vi "ApplyIVIConfigurationStore.vi"(8 "error in (no error)":errorcluster, 11 "Path":path) -> (0 "error out":errorcluster)   [LabVIEW 2009]
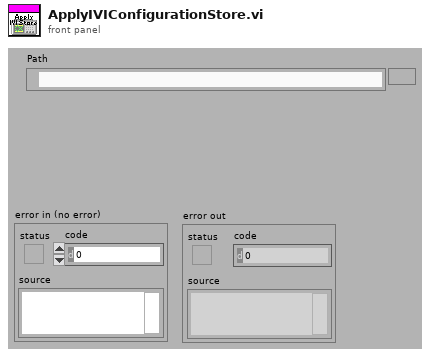
[diagram p1: front panel]
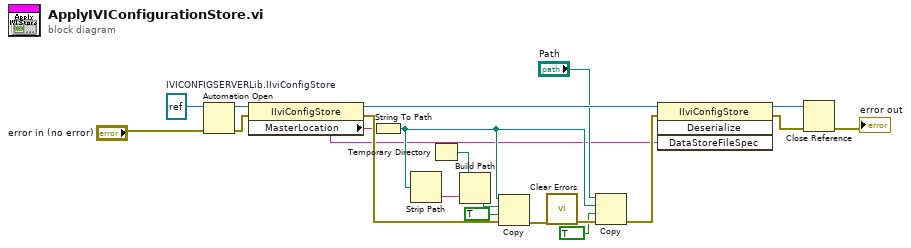
[diagram p0: block diagram]
diagram:
  w20 = refnum<k7> refnum  # IVICONFIGSERVERLib.IIviConfigStore
  n1 = Automation Open(error in (no error)="error in (no error)", Automation Refnum=w20) -> (Automation Refnum=w18:refnum<k7>, error out=w19:errorcluster)  [unwired: 2 out]
  n2 = property class="IIviConfigStore"(reference=w18, error in=w19) -> (reference out=w17:refnum<k7>, error out=w13:errorcluster, "MasterLocation"=w3:string)
  n3 = String To Path(string=w3) -> (path=w5:path)
  n4 = Strip Path(path=w5) -> (name=w15:string)  [unwired: 1 out]
  n5 = Temporary Directory() -> (w14:path)
  n6 = Build Path(base path=w14, name or relative path=w15) -> (appended path=w8:path)
  n7 = Copy(8:w13, 9:TRUE ("overwrite (F)"), 10:w8, 11:w5) -> (0:w16:errorcluster)  [unwired: 1 in, 2 out]
  n8 = call <vilib>:"Clear Errors.vi"("error in (no error)"=w16) -> ("error out"=w7:errorcluster)  [unwired: 6 in]
  n9 = Copy(8:w7, 9:TRUE ("overwrite (F)"), 10:w5, 11:"Path") -> (0:w4:errorcluster)  [unwired: 1 in, 2 out]
  n10 = invoke class="IIviConfigStore" method="Deserialize"(reference=w17, error in=w4, "DataStoreFileSpec"=w3) -> (reference out=w12:refnum<k7>, error out=w11:errorcluster)  [unwired: 1 in, 2 out]
  n11 = Close Reference(reference=w12, error in (no error)=w11) -> (error out=→"error out":errorcluster)
